vi "Get Class Control refnum incl if click on control.vi"(11 "Affected Items":T1) -> (1 "Class Name":string, 3 "RefNum out":refnum<vi>)   [LabVIEW 2023]
uses:
  top/BundleMagic.ctl
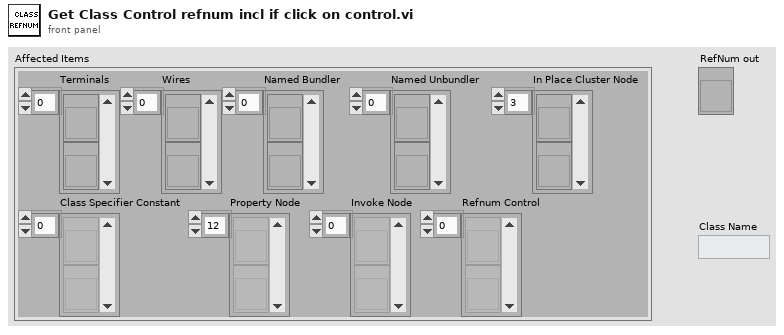
[diagram p1: front panel]
types:
  T1 = typedef "BundleMagic.ctl" = cluster{"Terminals":refnum<vi>[], "Wires":refnum<vi>[], "Named Bundler":refnum<vi>[], "Named Unbundler":refnum<vi>[], "In Place Cluster Node":refnum<vi>[], "Class Specifier Constant":refnum<vi>[], "Property Node":refnum<vi>[], "Invoke Node":refnum<vi>[], "Refnum Control":refnum<vi>[]}
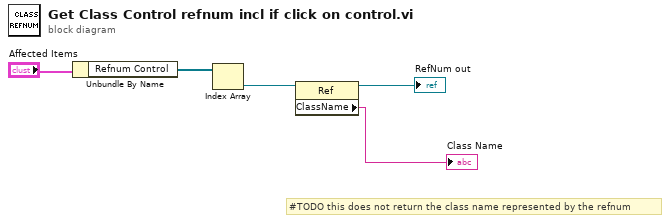
[diagram p0: block diagram]
diagram:
  # "#TODO this does not return the class name represented by the refnum"
  n1 = Unbundle By Name("Affected Items") -> ("Refnum Control"=w5:refnum<vi>[])
  n2 = Index Array(array=w5) -> (element=w4:refnum<vi>)  [unwired: 1 in]
  n3 = property class="Ref"(reference=w4) -> (reference out=→"RefNum out":refnum<vi>, "ClassName"=→"Class Name":string)  [unwired: 1 in, 1 out]
